vi "DELETEMAYBEstartIVSweepAndWait.vi"(8 "error in (no error)":errorcluster, 10 "Configure Sweep":T1 {"Channels"."Table" format="%#_1f"; "Channels"."Channel" min=1 max=128; "Channels"."Start" format="%#_6p"; "Channels"."End" format="%#_6p"; "Initial Wait (s)" format="%#_6p"}, 11 "Instrument.Lockin in":refnum<class "Instrument.Lockin.lvclass">) -> (0 "error out":errorcluster, 3 "Instrument.Lockin out":refnum<class "Instrument.Lockin.lvclass">)   [LabVIEW 2019, in "Instrument.Lockin.lvclass"]
uses:
  Instrument.Lockin.lvclass
  Instrument.DAQ/Typedefs/Sweep.Configuration--Cluster.ctl
  Instrument.DAQ/Instrument.DAQ.lvclass
  Instrument.DAQ/Typedefs/Sweep.Pattern--Enum.ctl
  Instrument.DAQ/Typedefs/Sweep.Channel--Cluster.ctl
  Instrument.DAQ/Typedefs/Sweep.Channel--Cluster--Array.ctl
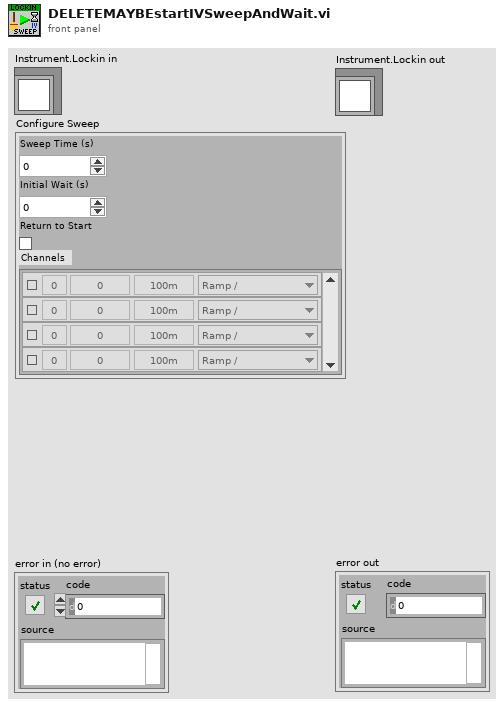
[diagram p1: front panel]
types:
  T1 = typedef "Instrument.DAQ.lvclass/Sweep.Configuration--Cluster.ctl" = cluster{"Sweep Time (s)":dbl, "Initial Wait (s)":dbl, "Return to Start":bool, "Channels":T2}
  T2 = typedef "Instrument.DAQ.lvclass/Sweep.Channel--Cluster--Array.ctl" = T3[]
  T3 = typedef "Instrument.DAQ.lvclass/Sweep.Channel--Cluster.ctl" = cluster{"Enable?":bool, "Channel":u16, "Start":dbl, "End":dbl, "Pattern":T4, "Table":dbl[]}
  T4 = typedef "Instrument.DAQ.lvclass/Sweep.Pattern--Enum.ctl" = enum16{"Ramp /", "Ramp /\\", "Smooth Ramp _/", "Smooth Ramp _/\\_", "Table"}
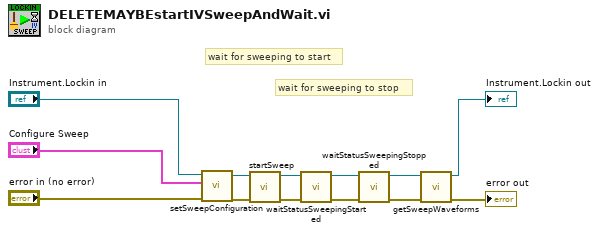
[diagram p0: block diagram]
diagram:
  # "wait for sweeping to stop"
  # "wait for sweeping to start"
  n1 = call-dynamic "setSweepConfiguration.vi"("error in (no error)"="error in (no error)", "Configure Sweep"="Configure Sweep", "Instrument.Lockin in"="Instrument.Lockin in") -> ("error out"=w9:errorcluster, "Instrument.Lockin out"=w10:refnum<class "Instrument.Lockin.lvclass">)  [unwired: 7 in]
  n2 = call-dynamic "startSweep.vi"("error in (no error)"=w9, "Instrument.Lockin in"=w10) -> ("error out"=w5:errorcluster, "Instrument.Lockin out"=w6:refnum<class "Instrument.Lockin.lvclass">)  [unwired: 8 in]
  n3 = call-dynamic "waitStatusSweepingStarted.vi"("error in (no error)"=w5, "Instrument.Lockin in"=w6) -> ("error out"=w4:errorcluster, "Instrument.Lockin out"=w7:refnum<class "Instrument.Lockin.lvclass">)  [unwired: 8 in]
  n4 = call "waitStatusSweepingStopped.vi"("error in (no error)"=w4, "Instrument.Lockin in"=w7) -> ("error out"=w3:errorcluster, "Instrument.Lockin out"=w2:refnum<class "Instrument.Lockin.lvclass">)  [unwired: 8 in]
  n5 = call-dynamic "getSweepWaveforms.vi"("error in (no error)"=w3, "Instrument.Lockin in"=w2) -> ("error out"=→"error out":errorcluster, "Instrument.Lockin out"=→"Instrument.Lockin out":refnum<class "Instrument.Lockin.lvclass">)  [unwired: 6 in, 2 out]
